vi "manual mode control.vi"(0 "X+":bool, 1 "Zs0":bool, 2 "X-":bool, 3 "Ys0":bool, 4 "Z+":bool, 6 "Y-":bool, 7 "Z-":bool, 8 "Y+":bool, 9 "HOME":bool, 10 "JOG FR":i8, 11 "RESET":bool, 13 "Xs0":bool) -> (14 "Send command":string, 15 "Valid command":bool)   [LabVIEW 2014, in "HPCNC.lvlib"]
uses:
  HPCNC.lvlib
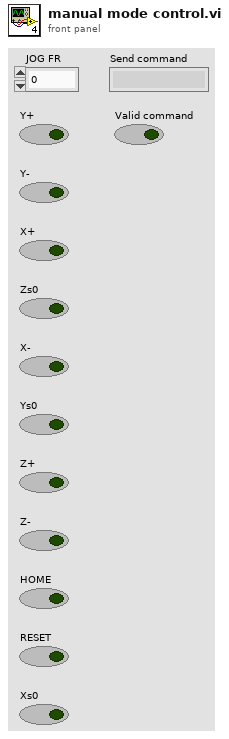
[diagram p1: front panel]
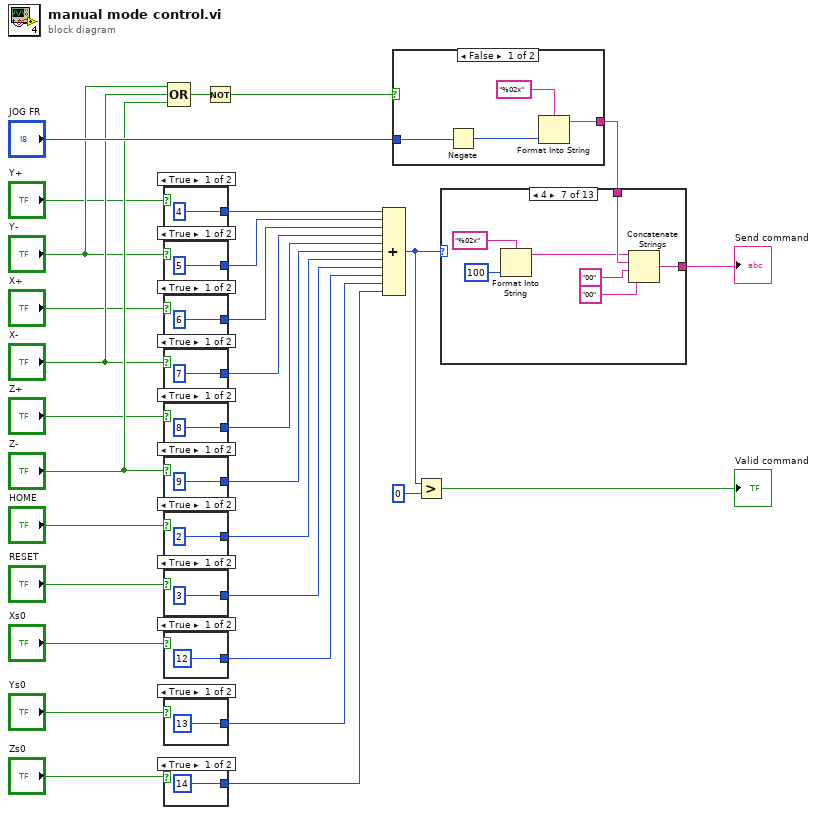
[diagram p0: block diagram]
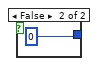
[diagram p2: hidden frame]
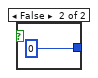
[diagram p3: hidden frame]
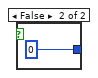
[diagram p4: hidden frame]
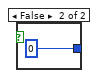
[diagram p5: hidden frame]
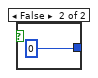
[diagram p6: hidden frame]
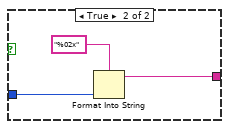
[diagram p7: hidden frame]
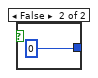
[diagram p8: hidden frame]
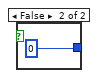
[diagram p9: hidden frame]
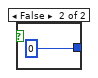
[diagram p10: hidden frame]
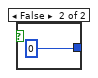
[diagram p11: hidden frame]
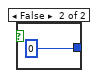
[diagram p12: hidden frame]
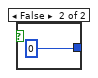
[diagram p13: hidden frame]
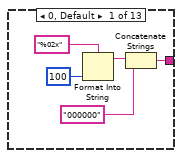
[diagram p14: hidden frame]
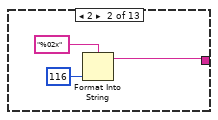
[diagram p15: hidden frame]
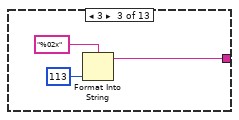
[diagram p16: hidden frame]
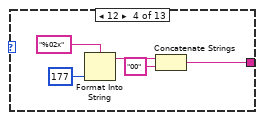
[diagram p17: hidden frame]
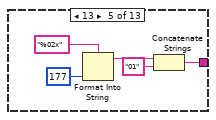
[diagram p18: hidden frame]
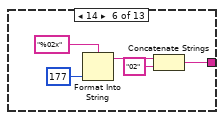
[diagram p19: hidden frame]
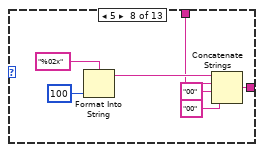
[diagram p20: hidden frame]
diagram:
  n1 = case shown="True" "Y+" {
    tunnel: [4 0] -> w1
    frame True {
    }
    frame False {
    }
  }
  n2 = case shown="True" "Y-" {
    tunnel: [5 0] -> w2
    frame True {
    }
    frame False {
    }
  }
  n3 = case shown="True" "X+" {
    tunnel: [6 0] -> w3
    frame True {
    }
    frame False {
    }
  }
  n4 = case shown="True" "X-" {
    tunnel: [7 0] -> w4
    frame True {
    }
    frame False {
    }
  }
  n5 = case shown="True" "Z+" {
    tunnel: [8 0] -> w5
    frame True {
    }
    frame False {
    }
  }
  n6 = case shown="True" "Z-" {
    tunnel: [9 0] -> w6
    frame True {
    }
    frame False {
    }
  }
  n7 = case shown="True" "HOME" {
    tunnel: [2 0] -> w14
    frame True {
    }
    frame False {
    }
  }
  n8 = case shown="True" "RESET" {
    tunnel: [3 0] -> w23
    frame True {
    }
    frame False {
    }
  }
  n9 = case shown="True" "Xs0" {
    tunnel: [12 0] -> w24
    frame True {
    }
    frame False {
    }
  }
  n10 = case shown="True" "Ys0" {
    tunnel: [13 0] -> w25
    frame True {
    }
    frame False {
    }
  }
  n11 = case shown="True" "Zs0" {
    tunnel: [14 0] -> w26
    frame True {
    }
    frame False {
    }
  }
  n12 = Compound Arithmetic op=OR("Y-", "X-", "Z-") -> (w10:bool)
  n13 = Not(x=w10) -> (.not. x?=w11:bool)
  n14 = Compound Arithmetic op=ADD(w1, w2, w3, w4, w5, w6, w14, w23, w24, w25, w26) -> (w7:i32)
  n15 = case shown="False" w11 {
    tunnel: "JOG FR" -> [w54 w59]
    tunnel: [w55 w57] -> w12
    frame False {
      n16 = Negate(x=w54) -> (-x=w53:i8)
      n17 = Format Into String(format string="%02x", w53) -> (resulting string=w55:string)  [unwired: 2 in, 1 out]
    }
    frame True {
      n18 = Format Into String(format string="%02x", w59) -> (resulting string=w57:string)  [unwired: 2 in, 1 out]
    }
  }
  n19 = Greater?(x=w7, y=0) -> (0:→"Valid command":bool)
  n20 = case shown="4" w7 {
    tunnel: w12 -> [_ _ _ _ _ _ w91 w94 w101 w107 w114 w121 _]
    tunnel: [w60 w65 w68 w71 w76 w81 w92 w93 w102 w108 w117 w124 "RESERVE"] -> w13
    frame 0, Default {
      n21 = Format Into String(format string="%02x", 100) -> (resulting string=w62:string)  [unwired: 2 in, 1 out]
      n22 = Concatenate Strings(w62, "000000" ("string")) -> (w60:string)
    }
    frame 2 {
      n23 = Format Into String(format string="%02x", 116) -> (resulting string=w65:string)  [unwired: 2 in, 1 out]
    }
    frame 3 {
      n24 = Format Into String(format string="%02x", 113) -> (resulting string=w68:string)  [unwired: 2 in, 1 out]
    }
    frame 12 {
      n25 = Format Into String(format string="%02x", 177) -> (resulting string=w73:string)  [unwired: 2 in, 1 out]
      n26 = Concatenate Strings(w73, "00" ("string")) -> (w71:string)
    }
    frame 13 {
      n27 = Format Into String(format string="%02x", 177) -> (resulting string=w78:string)  [unwired: 2 in, 1 out]
      n28 = Concatenate Strings(w78, "01" ("string")) -> (w76:string)
    }
    frame 14 {
      n29 = Format Into String(format string="%02x", 177) -> (resulting string=w83:string)  [unwired: 2 in, 1 out]
      n30 = Concatenate Strings(w83, "02" ("string")) -> (w81:string)
    }
    frame 4 {
      n31 = Format Into String(format string="%02x", 100) -> (resulting string=w86:string)  [unwired: 2 in, 1 out]
      n32 = Concatenate Strings(w86, w91, "00" ("string"), "00" ("string")) -> (w92:string)
    }
    frame 5 {
      n33 = Format Into String(format string="%02x", 100) -> (resulting string=w95:string)  [unwired: 2 in, 1 out]
      n34 = Concatenate Strings(w95, w94, "00" ("string"), "00" ("string")) -> (w93:string)
    }
    frame 6 {
      n35 = Format Into String(format string="%02x", 100) -> (resulting string=w103:string)  [unwired: 2 in, 1 out]
      n36 = Concatenate Strings(w103, "00" ("string"), w101, "00" ("string")) -> (w102:string)
    }
    frame 7 {
      n37 = Format Into String(format string="%02x", 100) -> (resulting string=w110:string)  [unwired: 2 in, 1 out]
      n38 = Concatenate Strings(w110, "00" ("string"), w107, "00" ("string")) -> (w108:string)
    }
    frame 8 {
      n39 = Format Into String(format string="%02x", 100) -> (resulting string=w118:string)  [unwired: 2 in, 1 out]
      n40 = Concatenate Strings(w118, "00" ("string"), "00" ("string"), w114) -> (w117:string)
    }
    frame 9 {
      n41 = Format Into String(format string="%02x", 100) -> (resulting string=w125:string)  [unwired: 2 in, 1 out]
      n42 = Concatenate Strings(w125, "00" ("string"), "00" ("string"), w121) -> (w124:string)
    }
    frame 11 {
    }
  }
  "Send command" <- w13
